vi "ATF Storage-AI_V_Scale_Config.vi"(8 "error in":errorcluster, 10 "AI C":T1(array[cluster]), 11 "task in":refnum<k21>) -> (0 "error out":errorcluster, 3 "task out":refnum<k21>)   [LabVIEW 2022 SP3]
uses:
  <vilib>/DAQmx/create/scale.llb/DAQmx Create Scale (Map Ranges).vi
  <vilib>/DAQmx/create/channels.llb/DAQmx Create Channel (AI-Voltage-Basic).vi
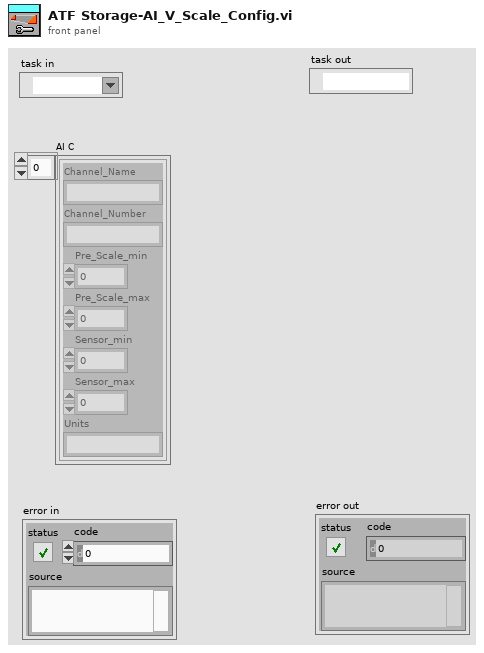
[diagram p1: front panel]
types:
  T1 = cluster{"Channel_Name":string, "Channel_Number":string, "Pre_Scale_min":dbl, "Pre_Scale_max":dbl, "Sensor_min":dbl, "Sensor_max":dbl, "Units":string}[]
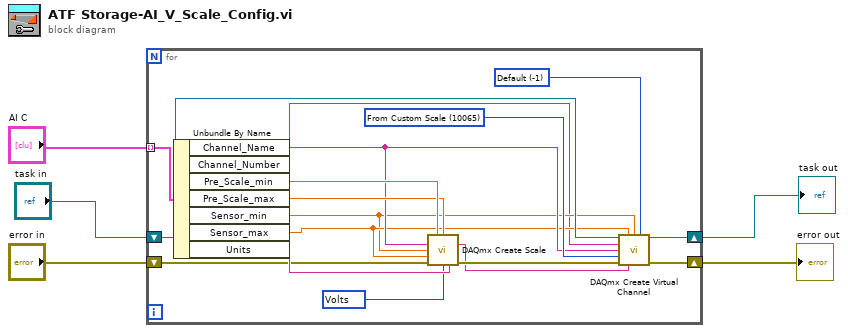
[diagram p0: block diagram]
diagram:
  n1 = for {
    tunnel: "AI C" -> [w22] mode=indexing
    shift-right: [w20] -> w2
    shift-left: "task in" -> [w21]
    shift-right: [w18] -> w3
    shift-left: "error in" -> [w10]
    w7 = 10348 items=["Volts"=10348, "Amps"=10342, "Deg F"=10144, "Deg C"=10143, "Deg R"=10145, "Kelvins"=10325, "Strain"=10299, "Ohms"=10384, "Hz"=10373, "Seconds"=10364, "Meters"=10219, "Inches"=10379, "Degrees"=10146, "Radians"=10273, "Ticks"=10304, "g"=10186, "m/s^2"=12470, "m/s"=15959, "in/s"=15960, "Pascals"=10081, "Newtons"=15875, "Pounds"=15876, "kgf"=15877, "psi"=15879, "bar"=15880, "Nm"=15881, "oz-in"=15882, "lb-in"=15883, "lb-ft"=15884, "Volts/Volt"=15896, "mVolts/Volt"=15897, "pCoulombs"=16103, "Coulombs"=16102, "From TEDS"=12516] ("pre-scaled units")
    w12 = 10065 items=["Volts"=10348, "From Custom Scale"=10065] ("units")
    w13 = -1 items=["Default"=-1, "RSE"=10083, "NRSE"=10078, "Differential"=10106, "Pseudodifferential"=12529] ("input terminal configuration")
    n2 = Unbundle By Name(w22) -> ("Channel_Name"=w11:string, "Channel_Number"=w6:string, "Pre_Scale_min"=w15:dbl, "Pre_Scale_max"=w14:dbl, "Sensor_min"=w8:dbl, "Sensor_max"=w9:dbl, "Units"=w17:string)
    n3 = call-poly <vilib>:"DAQmx Create Scale.vi"("pre-scaled minimum"=w15, "pre-scaled maximum"=w14, "name"=w11, "scaled minimum"=w8, "scaled maximum"=w9, "error in"=w10, "pre-scaled units"=w7, "scaled units"=w17) -> ("scale out"=w16:tag, "error out"=w19:errorcluster)  [unwired: 6 in]
    n4 = call-poly <vilib>:"DAQmx Create Virtual Channel.vi"("task in"=w21, "maximum value"=w9, "minimum value"=w8, "input terminal configuration"=w13, "physical channels"=w6, "name to assign"=w11, "units"=w12, "error in"=w19, "custom scale name"=w16) -> ("task out"=w20:refnum<k21>, "error out"=w18:errorcluster)  [unwired: 5 in]
  }
  "error out" <- w3
  "task out" <- w2
